vi "JAUS Reached waypoint.vi"(8 "Required distance to target (meters)":dbl, 9 "Number of WP Reached IN":i8, 10 "LocalPose in":T1, 11 "Local Waypoint List in":T3[](array[typedef])) -> (0 "Distance to Target (meters)":dbl=0.5, 1 "Number of WP Reached OUT":i8, 2 "Reached waypoint?":bool, 3 "Local Waypoint List Out":T3[](array[typedef]))   [LabVIEW 2009]
uses:
  JAUS/Support Files/ElementRec.ctl
  JAUS/Support Files/LocalWaypointRec.ctl
  JAUS/Support Files/LocalPose.ctl
  JAUS/Support Files/TimeRec.ctl
  Functional Global Variables/Actions for FG's.ctl
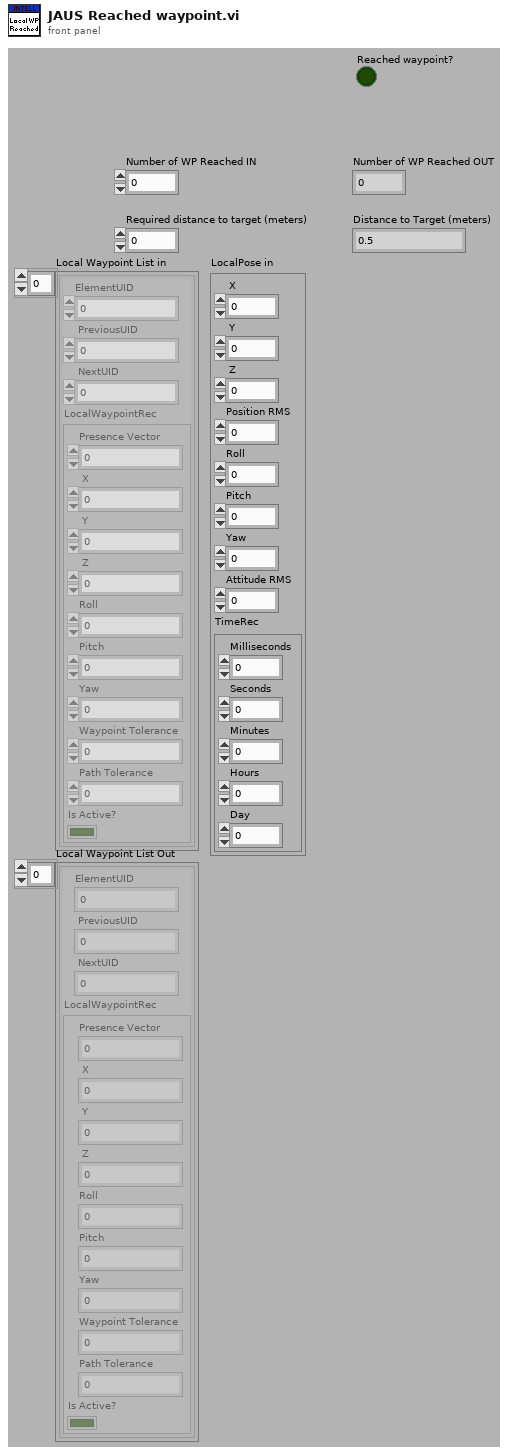
[diagram p1: front panel]
types:
  T1 = typedef "LocalPose.ctl" = cluster{" X":dbl, " Y":dbl, " Z":dbl, "Position RMS":dbl, "Roll":dbl, "Pitch":dbl, "Yaw":dbl, "Attitude RMS":dbl, "TimeRec":T2}
  T2 = typedef "TimeRec.ctl" = cluster{"Milliseconds":u32, "Seconds":u32, "Minutes":u32, "Hours":u32, "Day":u32}
  T3 = typedef "ElementRec.ctl" = cluster{"ElementUID":u16, " PreviousUID":u16, " NextUID":u16, "LocalWaypointRec":T4}
  T4 = typedef "LocalWaypointRec.ctl" = cluster{"Presence Vector":u8, " X":dbl, " Y":dbl, " Z":dbl, "Roll":dbl, "Pitch":dbl, "Yaw":dbl, "Waypoint Tolerance":dbl, "Path Tolerance":dbl, "Is Active?":bool}
  T5 = typedef "Actions for FG's.ctl" = enum16{"Read", "Write"}
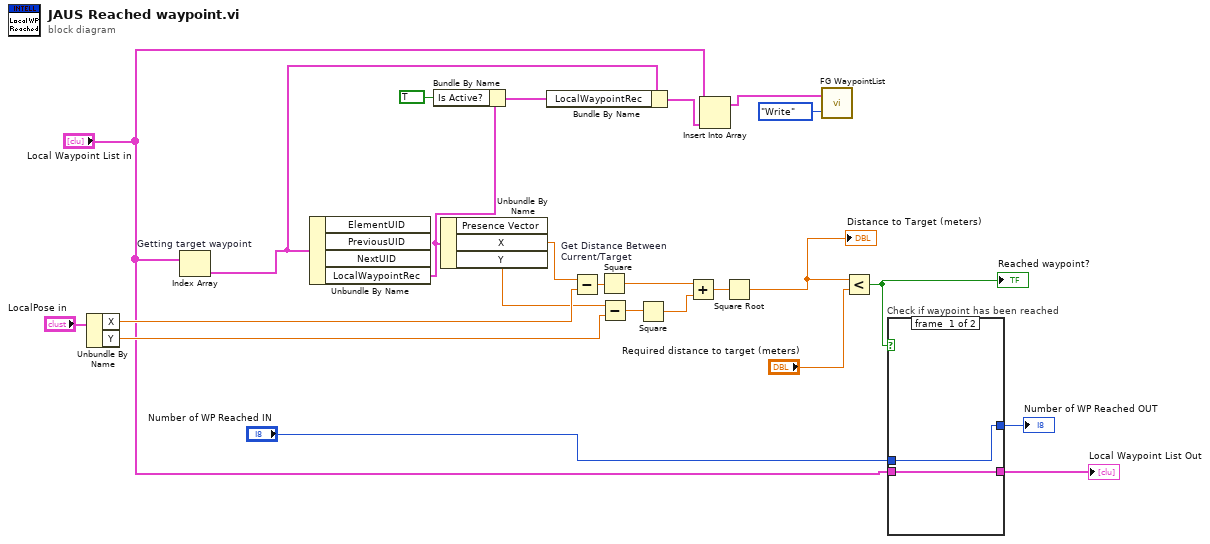
[diagram p0: block diagram]
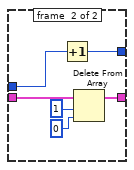
[diagram p2: hidden frame]
diagram:
  n1 = Unbundle By Name("LocalPose in") -> ("X"=w17:dbl, "Y"=w15:dbl)
  n2 = Index Array "Getting target waypoint"(array="Local Waypoint List in") -> (element=w5:T3)  [unwired: 1 in]
  n3 = Unbundle By Name(w5) -> ("LocalWaypointRec"=w7:T4)  [unwired: 3 out]
  n4 = Bundle By Name(cluster=w7, "Is Active?"=TRUE) -> (w4:T4)
  n5 = Unbundle By Name(w7) -> ("X"=w18:dbl, "Y"=w16:dbl)  [unwired: 1 out]
  n6 = Bundle By Name(cluster=w5, "LocalWaypointRec"=w4) -> (w2:T3)
  n7 = Subtract(x=w18, y=w17) -> (x-y=w14:dbl)
  n8 = Square "Get Distance Between Current/Target"(x=w14) -> (x^2=w12:dbl)
  n9 = Subtract(x=w16, y=w15) -> (x-y=w13:dbl)
  n10 = Square(x=w13) -> (x^2=w11:dbl)
  n11 = Add(x=w12, y=w11) -> (x+y=w10:dbl)
  n12 = Insert Into Array(array="Local Waypoint List in", new element=w2) -> (w1:T3[])  [unwired: 1 in]
  n13 = Square Root(x=w10) -> (sqrt(x)=w9:dbl)
  "Distance to Target (meters)" <- w9
  n14 = call "FG WaypointList.vi"("FG Action (Read)"=Actions_for_FG's."Write", "Local Waypoint List in"=w1) -> ()  [unwired: 1 out]
  n15 = Less?(x=w9, y="Required distance to target (meters)") -> (x < y?=w24:bool)
  "Reached waypoint?" <- w24
  n16 = case "Check if waypoint has been reached" shown="True" w24 {
    tunnel: "Local Waypoint List in" -> [w26 w32]
    tunnel: [w26 w29] -> w20
    tunnel: [w25 w28] -> w22
    tunnel: "Number of WP Reached IN" -> [w25 w27]
    frame #0 {
    }
    frame #1 {
      n17 = Increment(x=w27) -> (x+1=w28:i8)
      n18 = Delete From Array(array=w32, length=1, index=0) -> (array with subset deleted=w29:T3[])  [unwired: 1 out]
    }
  }
  "Number of WP Reached OUT" <- w22
  "Local Waypoint List Out" <- w20
